vi "Delete Uint8Array DVR.vi"(8 "error in (no error)":errorcluster, 11 "Uint8Array DVR in":refnum<data-value>) -> (0 "error out":errorcluster, 3 "Uint8Array out":refnum<class "Uint8Array.lvclass">)   [LabVIEW 2012, in "MDSplus.lvlib" / "Uint8Array.lvclass"]
uses:
  <vilib>/MDSplus/Classes/Data_Class/Array_Class/Uint8Array_Class/Uint8Array.lvclass
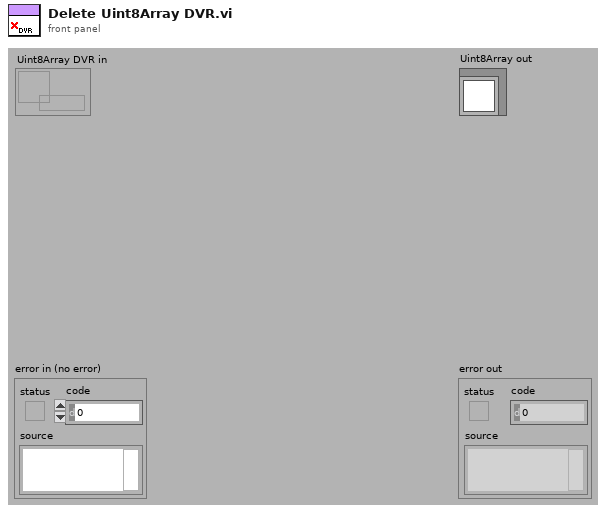
[diagram p1: front panel]
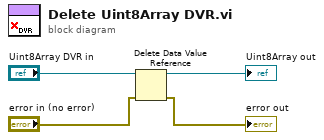
[diagram p0: block diagram]
diagram:
  n1 = Delete Data Value Reference(data value reference="Uint8Array DVR in", error in="error in (no error)") -> (data value=→"Uint8Array out":refnum<class "Uint8Array.lvclass">, error out=→"error out":errorcluster)
